vi "BRig_dataTrial_Cue2_iCue_Low.vi"() -> (2 "output_Cue2_iCue_Low":i32)   [LabVIEW 2014]
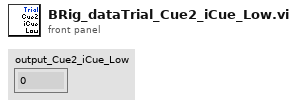
[diagram p1: front panel]
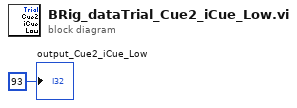
[diagram p0: block diagram]
diagram:
  "output_Cue2_iCue_Low" <- 93 ("output_iBlock")
